vi "Test Fail Lamp.vi"   [LabVIEW 2020]
types:
  T1 = enum16{"Reset", "Yellow Lamp&Alarm", "Green Lamp&Alarm", "Red Lamp&Alarm"}
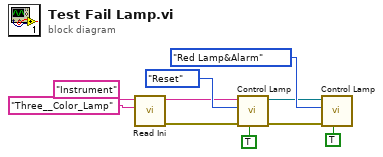
[diagram p0: block diagram]
diagram:
  n1 = call "Read Ini.vi"("key"="Three__Color_Lamp", "section"="Instrument") -> ("error out"=w4:errorcluster, "value"=w2:string)  [unwired: 8 in]
  n2 = call "Control Lamp.vi"("Lamp State"=TRUE, "error in (no error)"=w4, "Function Choose"=T1."Reset", "VISA resource name"=w2) -> ("error out"=w3:errorcluster, "VISA resource name out"=w1:refnum<visa-resource-name>)  [unwired: 6 in]
  n3 = call "Control Lamp.vi"("Lamp State"=TRUE, "error in (no error)"=w3, "Function Choose"=T1."Red Lamp&Alarm", "VISA resource name"=w1) -> ()  [unwired: 6 in, 2 out]
